vi "Build Param Properties.vi"(0 "ARINC Parameter":T1, 5 "error in (no error)":errorcluster) -> (7 "signed":bool, 8 "Prop Names":string[](array[string]), 9 "numberBits":i32, 10 "Prop Values":variant[](array[variant]), 11 "startBit":i32, 13 "scaleFactor":dbl, 16 "name":string, 18 "error out":errorcluster, 19 "scaleOffset":dbl)   [LabVIEW 2015, in "AIT 429 System Explorer.lvlib"]
uses:
  AIT 429 System Explorer.lvlib
  Controls/ARINCParam.ctl
  Shared/Controls and Global/Global.vi
  Shared/AIT 429 Shared.lvlib
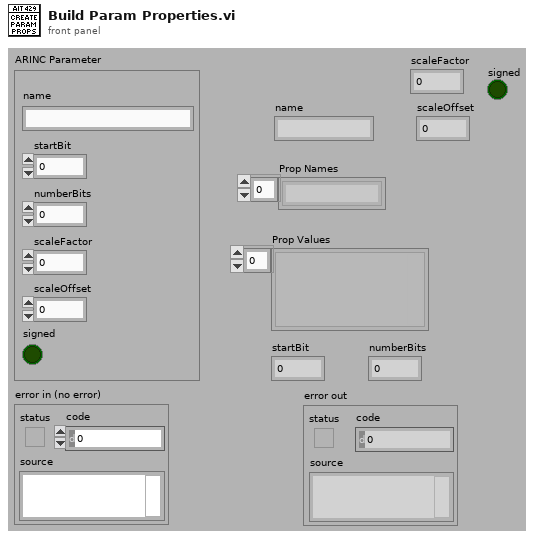
[diagram p1: front panel]
types:
  T1 = typedef "AIT 429 System Explorer.lvlib/ARINCParam.ctl" = cluster{"name":string, "startBit":i32, "numberBits":i32, "scaleFactor":dbl, "scaleOffset":dbl, "signed":bool}
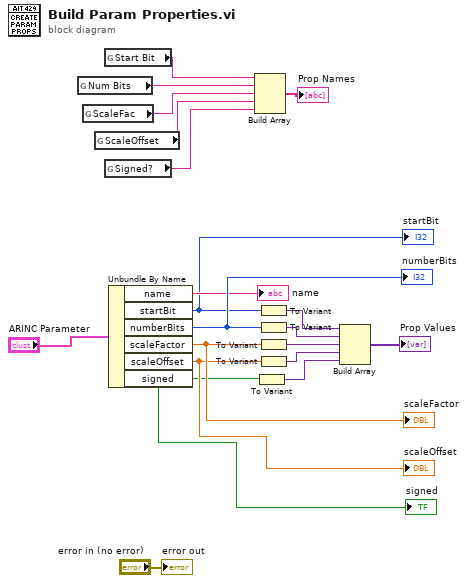
[diagram p0: block diagram]
diagram:
  n1 = global read "Global.vi" "Num Bits"() -> (w13:string)
  n2 = global read "Global.vi" "ScaleFac"() -> (w11:string)
  n3 = global read "Global.vi" "ScaleOffset"() -> (w5:string)
  n4 = global read "Global.vi" "Start Bit"() -> (w12:string)
  n5 = global read "Global.vi" "Signed?"() -> (w4:string)
  n6 = Unbundle By Name("ARINC Parameter") -> ("name"=→"name":string, "startBit"=w14:i32, "numberBits"=w19:i32, "scaleFactor"=w8:dbl, "scaleOffset"=w7:dbl, "signed"=w3:bool)
  "startBit" <- w14
  "numberBits" <- w19
  "scaleOffset" <- w7
  "scaleFactor" <- w8
  "signed" <- w3
  n7 = Build Array(w12, w13, w11, w5, w4) -> (→"Prop Names":string[])
  n8 = To Variant(anything=w3) -> (Variant=w2:variant)
  n9 = To Variant(anything=w14) -> (Variant=w17:variant)
  n10 = To Variant(anything=w19) -> (Variant=w16:variant)
  n11 = To Variant(anything=w8) -> (Variant=w10:variant)
  n12 = To Variant(anything=w7) -> (Variant=w6:variant)
  n13 = Build Array(w17, w16, w10, w6, w2) -> (→"Prop Values":variant[])
  "error out" <- "error in (no error)"
